vi "week04_Ex02.vi"() -> ()   [LabVIEW 2017]
panel:
  out "all lower case string":string
  in  "String":string
  out "substring":string
  out "length":i32
  in  "string":string
  out "Round":i32
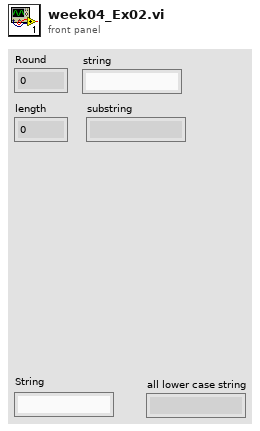
[diagram p1: front panel]
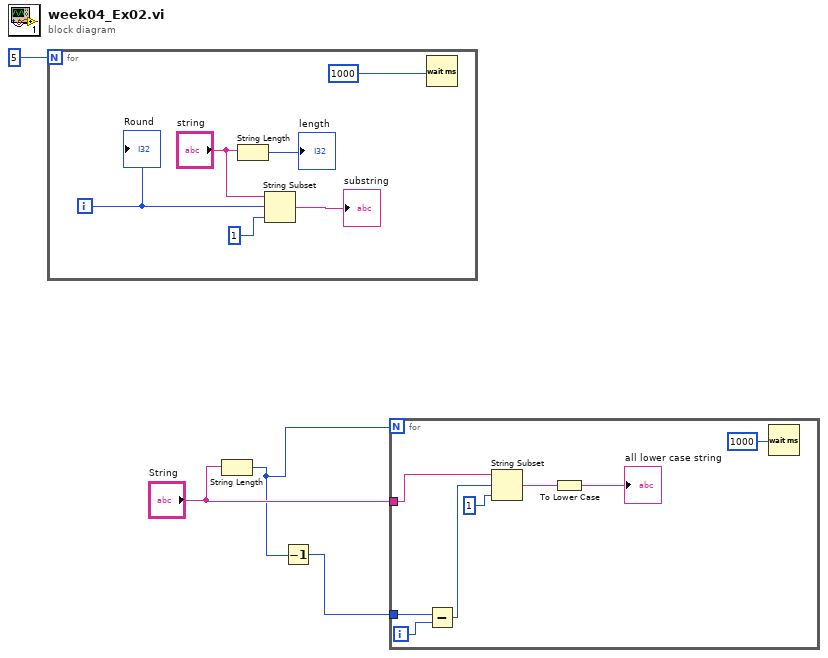
[diagram p0: block diagram]
diagram:
  n1 = for {
    N: 5 -> [_]
    i -> [w5]
    n2 = String Length(string="string") -> (length=→"length":i32)
    n3 = String Subset(string="string", offset (0)=w5, length (rest)=i8 1 ("length (rest)")) -> (substring=→"substring":string)
    n4 = Wait (ms)(milliseconds to wait=u32 1000) -> ()  [unwired: 1 out]
    "Round" <- w5
  }
  n5 = String Length(string="String") -> (length=w2:i32)
  n6 = Decrement(x=w2) -> (x-1=w1:i32)
  n7 = for {
    N: w2 -> [_]
    tunnel: "String" -> [w14]
    tunnel: w1 -> [w11]
    i -> [w13]
    n8 = Subtract(x=w11, y=w13) -> (x-y=w12:i32)
    n9 = String Subset(string=w14, offset (0)=w12, length (rest)=1 ("length (rest)")) -> (substring=w15:string)
    n10 = To Lower Case(string=w15) -> (all lower case string=→"all lower case string":string)
    n11 = Wait (ms)(milliseconds to wait=u32 1000) -> ()  [unwired: 1 out]
  }
